vi "LAUDA_CONTROL07.vi"(0 "Bypass":bool, 1 "PAUSE":bool, 2 "data":dynamicdata(waveform), 3 "Seq":dbl[][](array[numeric])=[[20.0, 45.0, 50.0], [46.0, 50.0, 20.0], [3.0, 3.0, 3.0]], 4 "Lauda port":dbl=9.0, 5 "Tbypass":dbl=20.0, 6 "Treshold":dbl, 7 "Bypass select":enum32{"Tr", "Tj"}(radio), 8 "err":i32, 9 "Shutdown":bool, 10 "Master Start":bool, 11 "Reset":bool, 13 "Tfail (manual)":dbl, 15 "Tmax":dbl, 26 "T ext / T ext 2":enum32{"External 1", "External 2"}(radio), 27 "Tmin":dbl) -> (12 "Tj in":dbl, 14 "DT":dbl, 16 "Tj out":dbl, 17 "Tset":dbl, 18 "Dynamic Data":dynamicdata(waveform), 19 "T ext 2":dbl, 20 "Numeric":i16, 21 "Numeric 2":dbl, 22 "T control":dbl, 23 "Current step":i32, 24 "Elapsed":i32, 25 "Tr":dbl)   [LabVIEW 2015]
uses:
  x64/Debug/BERTTA.dll
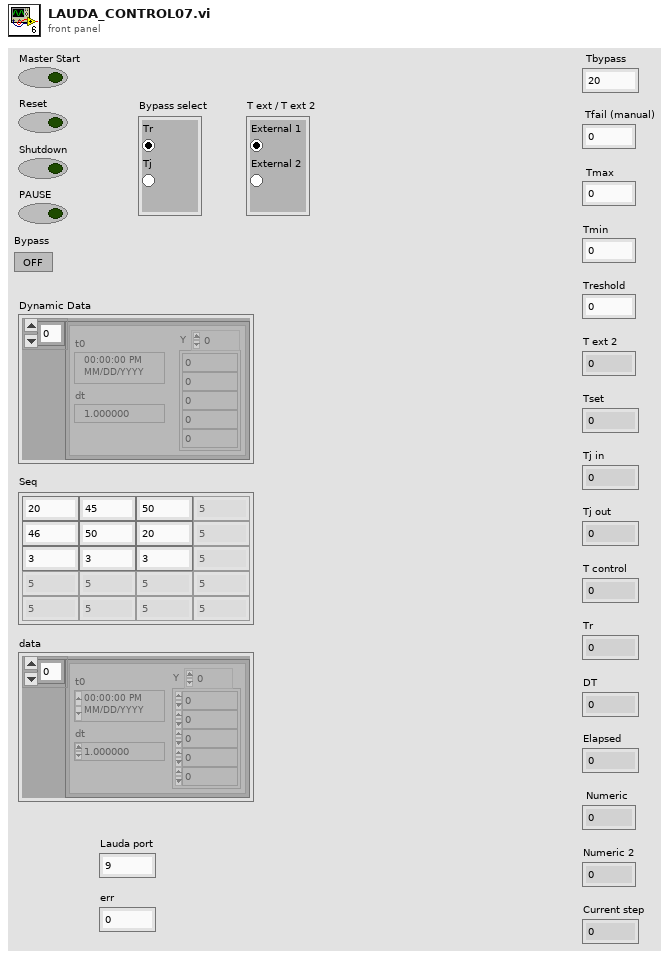
[diagram p1: front panel]
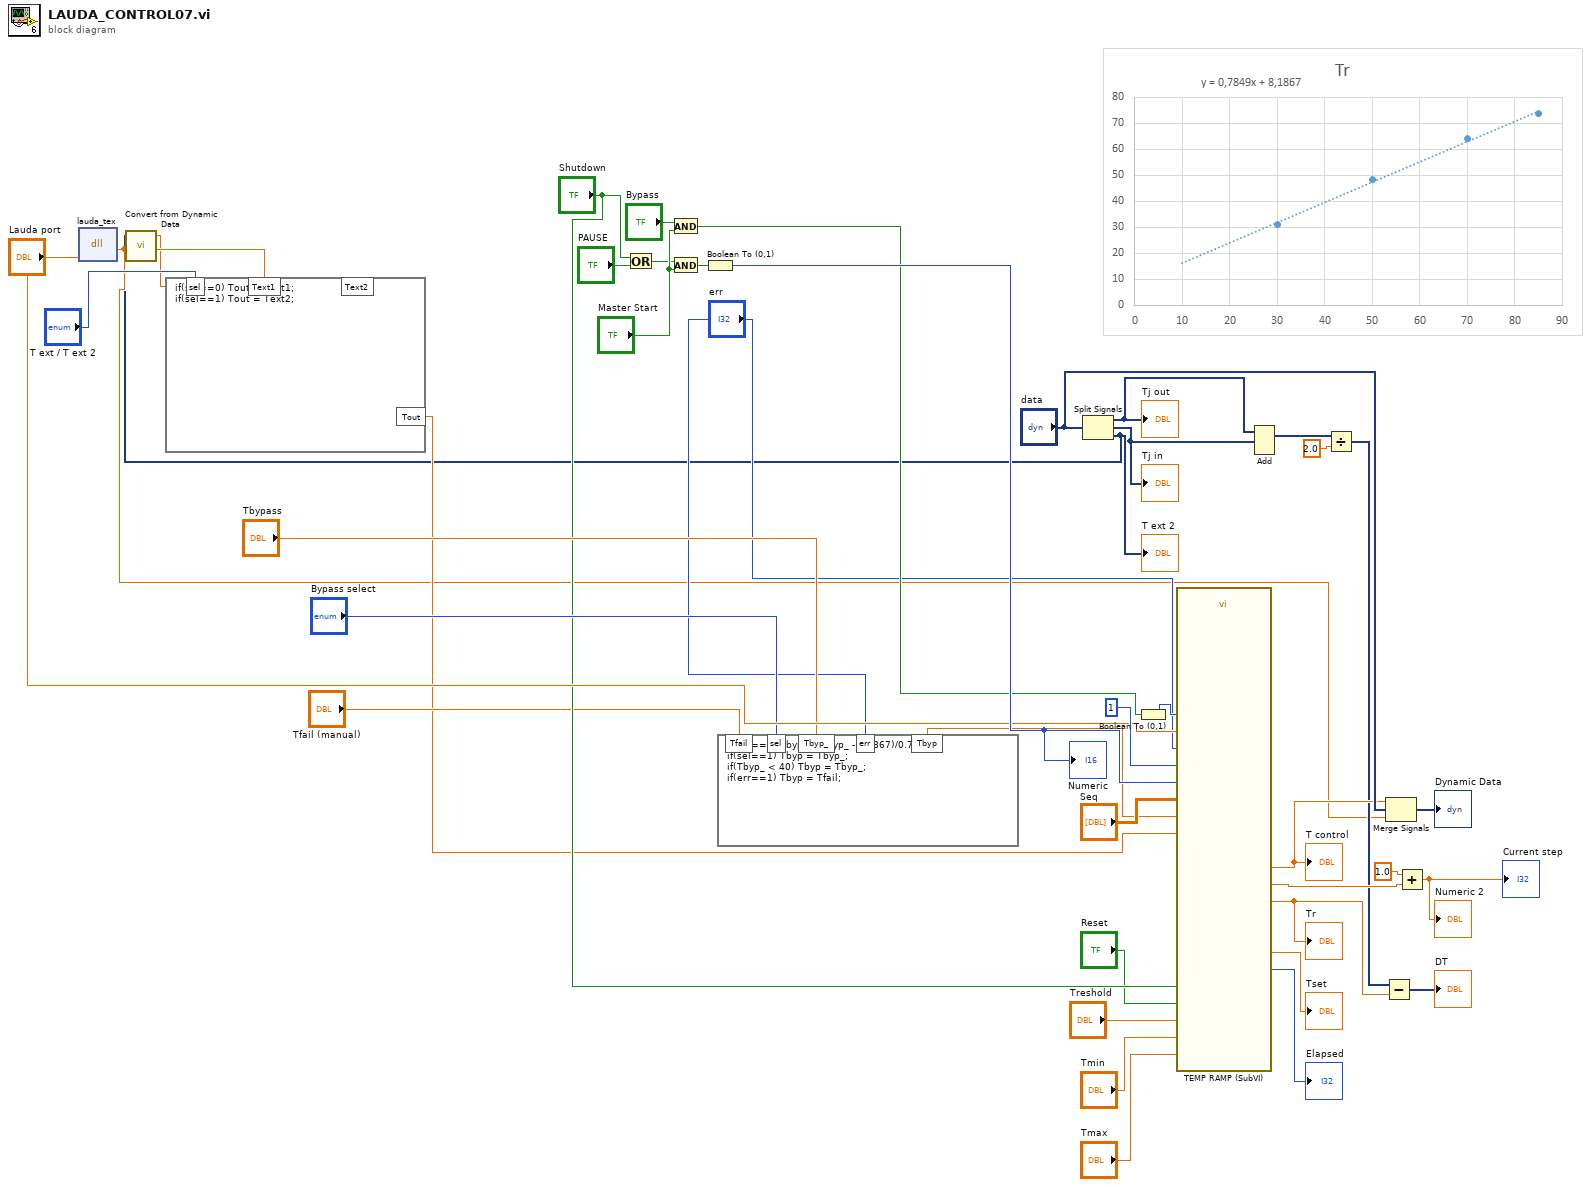
[diagram p0: block diagram]
diagram:
  n1 = dll-call lib="C:/Users/shresplab/OneDrive - Kemira Oyj/Documents/Visual Studio 2017/Projects/Bertta/BERTTA/x64/Debug/BERTTA.dll" fn="lauda_tex"("port"="Lauda port") -> ("return type"=w3:dbl)  [unwired: 4 in, 2 out]
  n2 = Or(x="Shutdown", y="PAUSE") -> (x .or. y?=w19:bool)
  n3 = And(x="Bypass", y="Master Start") -> (x .and. y?=w22:bool)
  n4 = And(x=w19, y="Master Start") -> (x .and. y?=w40:bool)
  n5 = Boolean To (0,1)(Boolean=w40) -> (0, 1=w36:i16)
  "Numeric" <- w36
  n6 = formula code="if(sel==0) Tbyp = (Tbyp_ - 8.1867)/0.7849;\nif(sel==1) Tbyp = Tbyp_;\nif(Tbyp_ < 40) Tbyp = Tbyp_;\nif(err==1) Tbyp = Tfail;"("Tbyp_"="Tbypass", "sel"="Bypass select", "Tfail"="Tfail (manual)", "err"="err") -> ("Tbyp"=w24:dbl)
  n7 = Split Signals("data") -> (w39:dynamicdata, w38:dynamicdata, w2:dynamicdata)  [unwired: 3 in]
  "Tj in" <- w38
  "Tj out" <- w39
  "T ext 2" <- w2
  n8 = call "Convert from Dynamic Data"("Dynamic Data Type"=w2) -> ("Scalar"=w1:dbl)  [unwired: 3 in]
  n9 = formula code="if(sel==0) Tout = Text1;\nif(sel==1) Tout = Text2;"("sel"="T ext / T ext 2", "Text1"=w3, "Text2"=w1) -> ("Tout"=w4:dbl)
  n10 = Boolean To (0,1)(Boolean=w22) -> (0, 1=w28:i16)
  n11 = call "TEMP RAMP (SubVI).vi"("Device port"="Lauda port", "enable"=i16 1 ("Numeric"), "Tbyp"=w24, "pause"=w36, "Seq"="Seq", "Tcurrent"=w4, "bypass"=w28, "T_low"="Tmin", "T_up"="Tmax", "err"="err", "Treshold"="Treshold", "Reset"="Reset", "Shutdown"="Shutdown") -> ("Step out"=w33:dbl, "T"=w10:dbl, "Sp"=w30:dbl, "elapsed"=→"Elapsed":i32, "Tset"=→"Tset":dbl)  [unwired: 7 in, 3 out]
  "T control" <- w30
  "Tr" <- w10
  n12 = Add(1:w38, 2:w39) -> (0:w14:dynamicdata)  [unwired: 1 in, 1 out]
  n13 = Divide(x=w14, y=2.0) -> (x/y=w11:dynamicdata)
  n14 = Subtract(x=w11, y=w10) -> (x-y=→"DT":dynamicdata)
  n15 = Merge Signals(w30, "data", w3) -> (→"Dynamic Data":dynamicdata)
  n16 = Add(x=1.0, y=w33) -> (x+y=→"Current step" →"Numeric 2":dbl)
